vi "HeatFlow Acquire.vi"(0 "HeatFlow HW Tasks in":T4, 1 "HeatFlow HW Cfg":T1, 2 "Runtime":T3, 3 "Last element?":bool) -> (7 "Log Stream":T2, 9 "Display Stream":T2, 10 "error out":errorcluster)   [LabVIEW 2019, in "Acquisition.lvlib"]
doc: "Perform the acquisition. Replace the contents of this diagram with calls to acquisition hardware."
uses:
  Acquisition.lvlib
  HeatFlow HW Tasks.ctl
  Settings/Runtime Conf.ctl
  <extravilib>/ChannelInstances/Stream-var/)Channel.ctl
  HeatFlow HW Cfg.ctl
  HeatFlow Acq Data.ctl
  HeatFlow Acq States.ctl
  <vilib>/DAQmx/read.llb/DAQmx Read (Analog 1D DBL NChan 1Samp).vi
  <vilib>/DAQmx/write.llb/DAQmx Write (Analog 1D DBL NChan 1Samp).vi
  <vilib>/DAQmx/read.llb/DAQmx Read (Analog DBL 1Chan 1Samp).vi
  <extravilib>/ChannelInstances/Stream-var/Write With Abort.vi
  <extravilib>/ChannelInstances/Stream-var/Endpoint.vi
  <vilib>/DAQmx/miscellaneous.llb/DAQmx Fill In Error Info.vi
  <extravilib>/ChannelInstances/Stream-var/)Channel.vi
  <resource>/ChannelSupport/_ChannelSupport/WaitIfNeeded.vi
  <extravilib>/ChannelInstances/Stream-var.lvlib
  Settings/Settings.lvlib
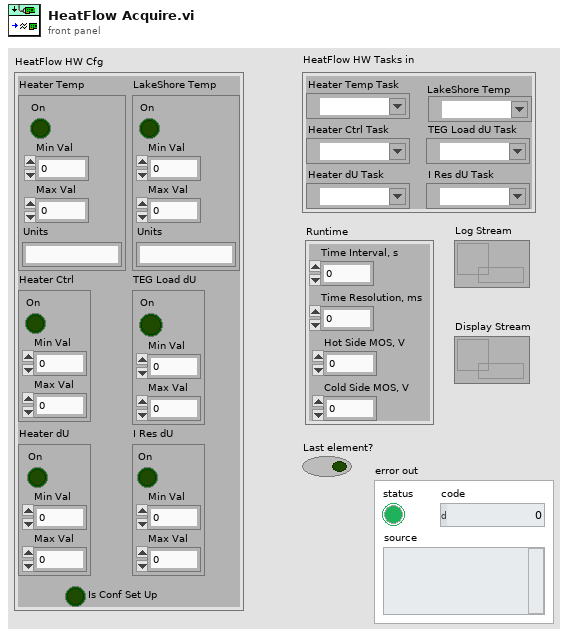
[diagram p1: front panel]
types:
  T1 = typedef "Acquisition.lvlib/HeatFlow HW Cfg.ctl" = cluster{"Heater Temp":cluster{"On":bool, "Min Val":dbl, "Max Val":dbl, "Units":string}, "LakeShore Temp":cluster{"On":bool, "Min Val":dbl, "Max Val":dbl, "Units":string}, "Heater Ctrl":cluster{"On":bool, "Min Val":dbl, "Max Val":dbl}, "TEG Load dU":cluster{"On":bool, "Min Val":dbl, "Max Val":dbl}, "Heater dU":cluster{"On":bool, "Min Val":dbl, "Max Val":dbl}, "I Res dU":cluster{"On":bool, "Min Val":dbl, "Max Val":dbl}, "Is Conf Set Up":bool}
  T2 = typedef "Stream-var.lvlib/)Channel.ctl" = refnum<queue>
  T3 = typedef "Settings.lvlib/Runtime Conf.ctl" = cluster{"Time Interval, s":dbl, "Time Resolution, ms":u32, "Hot Side MOS, V":dbl, "Cold Side MOS, V":dbl}
  T4 = typedef "Acquisition.lvlib/HeatFlow HW Tasks.ctl" = cluster{"Heater Temp Task":refnum<k21>, "Heater Ctrl Task":refnum<k21>, "TEG Load dU Task":refnum<k21>, "Heater dU Task":refnum<k21>, "I Res dU Task":refnum<k21>, "LakeShore Temp":refnum<visa-resource-name>}
  T5 = typedef "Acquisition.lvlib/HeatFlow Acq Data.ctl" = cluster{"Time Stamp":timestamp, "Time Delta":u32, "LakeShore_Temp":cluster{"Tube_T_1":dbl, "Tube_T_2":dbl, "Tube_T_3":dbl, "Tube_T_4":dbl, "Tube_T_5":dbl, "Tube_T_6":dbl, "Tube_T_7":dbl, "Tube_T_8":dbl}, "Heaters":cluster{"I_Res_dU":dbl, "Heater_dU":dbl, "Hot_Side_I":dbl, "Hot_Side_P":dbl, "Cold_Ctrl_U":dbl, "Hot_Ctrl_U":dbl, "Hot_Side_T":dbl, "Cold_Side_T":dbl}, "TEG":cluster{"TEG_Load_dU":dbl, "TEG_Load_R":dbl, "TEG_Load_I":dbl, "TEG_Load_P":dbl, "TEG_eta":dbl, "TEG_dT":dbl, "TEG_U_open":dbl, "TEG_U_Test":dbl, "TEG_R_Test":dbl, "TEG_Rw":dbl}, "LastElement?":bool}
  T6 = typedef "Acquisition.lvlib/HeatFlow Acq States.ctl" = enum16{"Start", "--- Control ---", "HeaterTemp", "DoControl?", "HeaterCtrl", "--- Readings ---", "DoReadings?", "I_Res_dU", "LakeShoreTemp", "Heater_dU", "TEG_Load_dU", "Calculations", "End"}
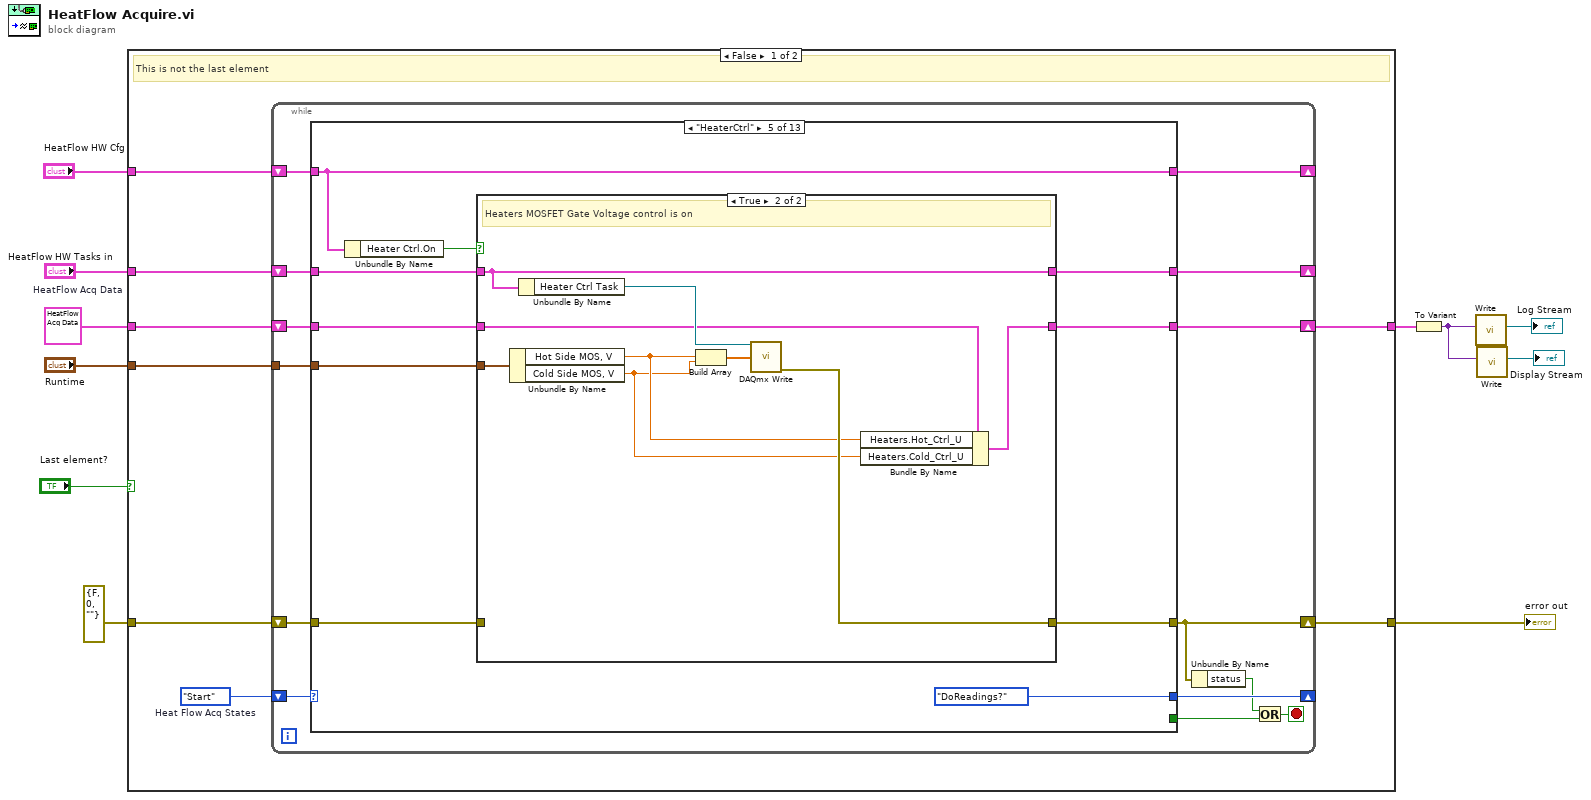
[diagram p0: block diagram]
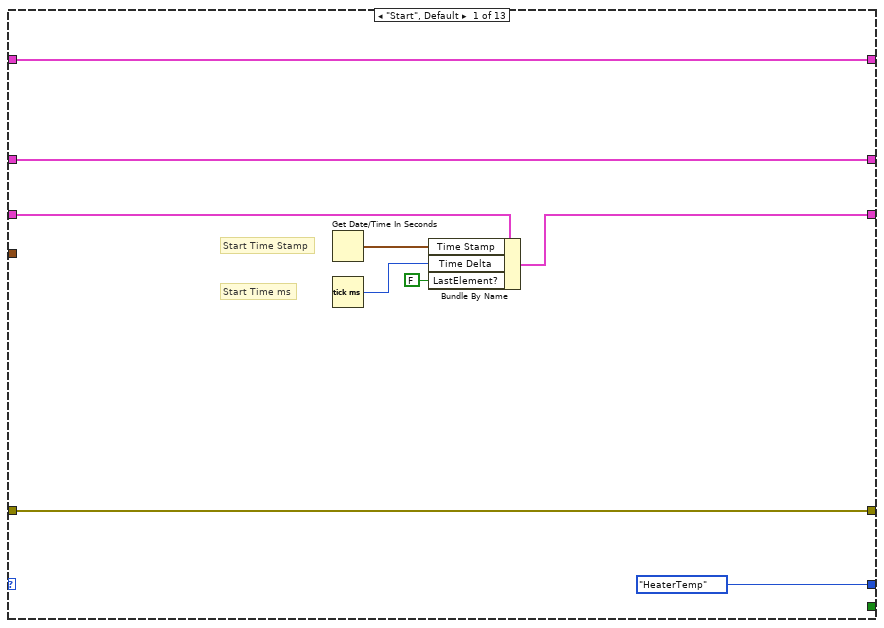
[diagram p2: hidden frame]
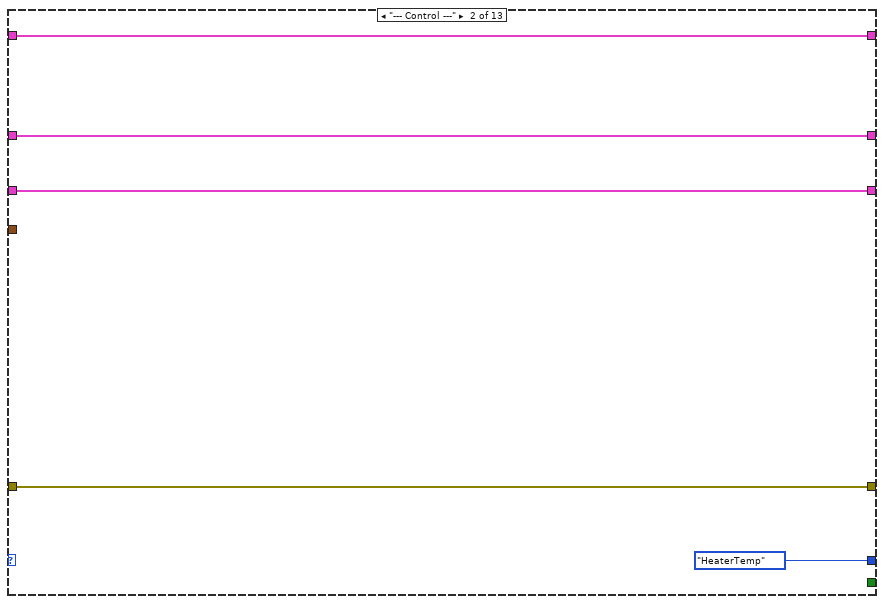
[diagram p3: hidden frame]
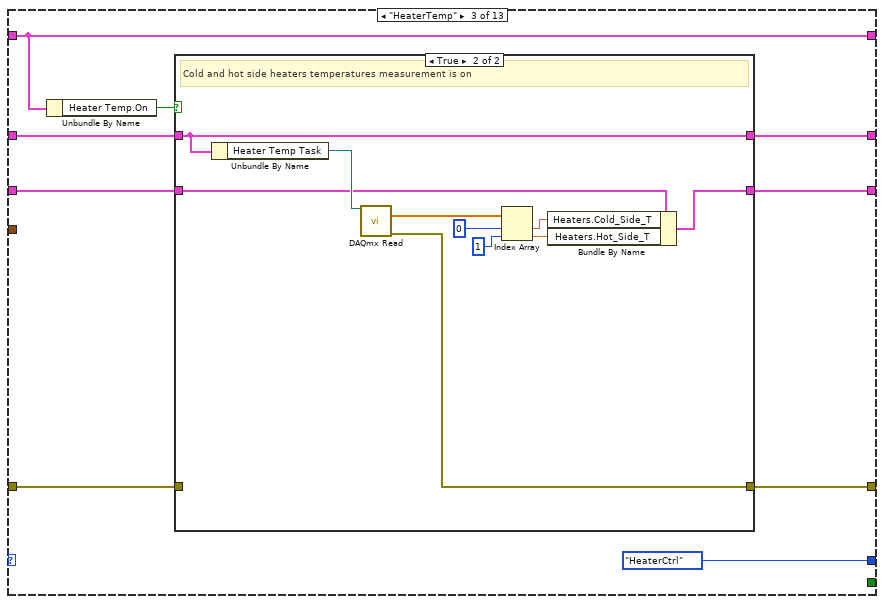
[diagram p4: hidden frame]
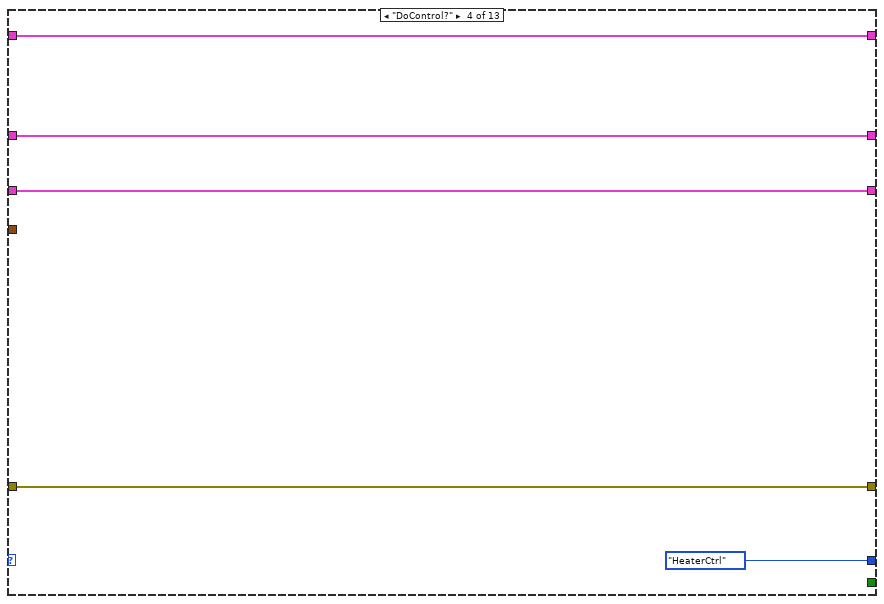
[diagram p6: hidden frame]
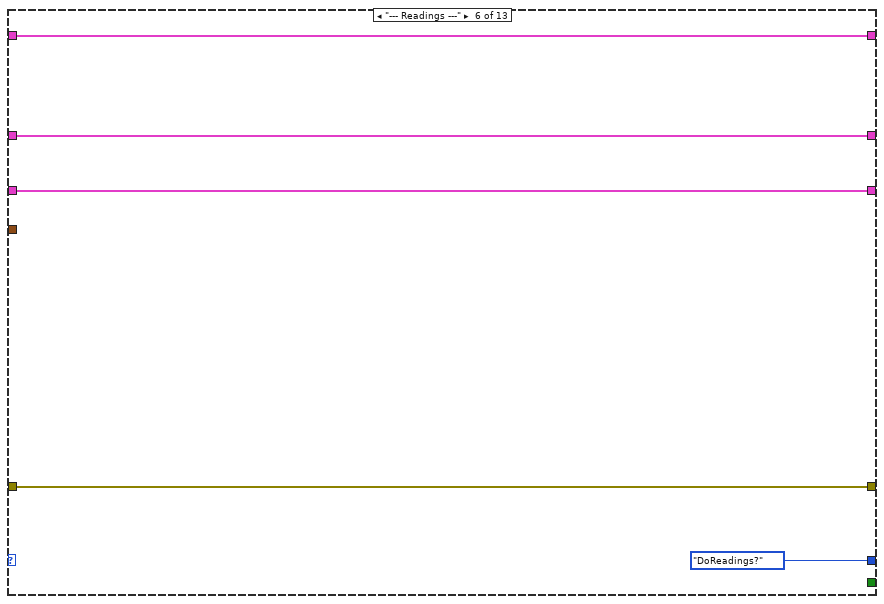
[diagram p8: hidden frame]
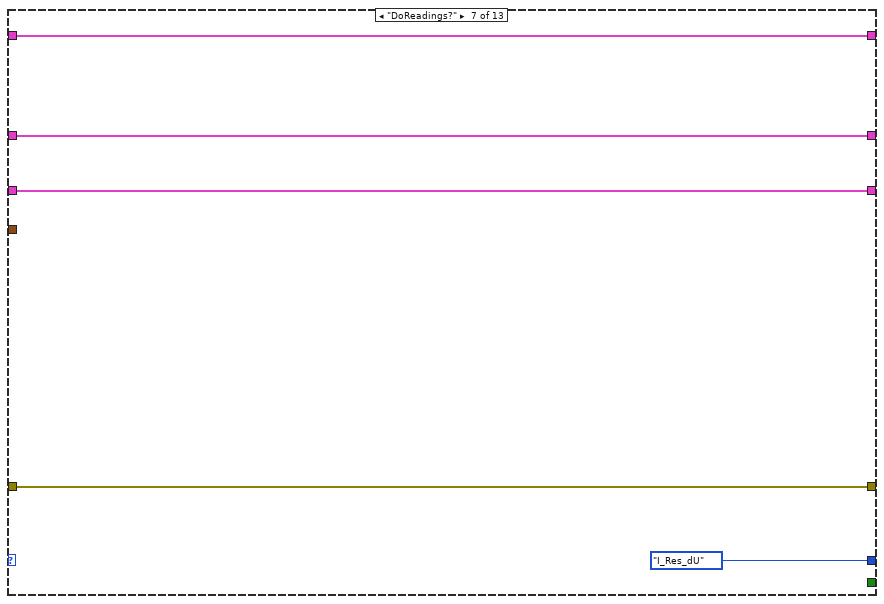
[diagram p9: hidden frame]
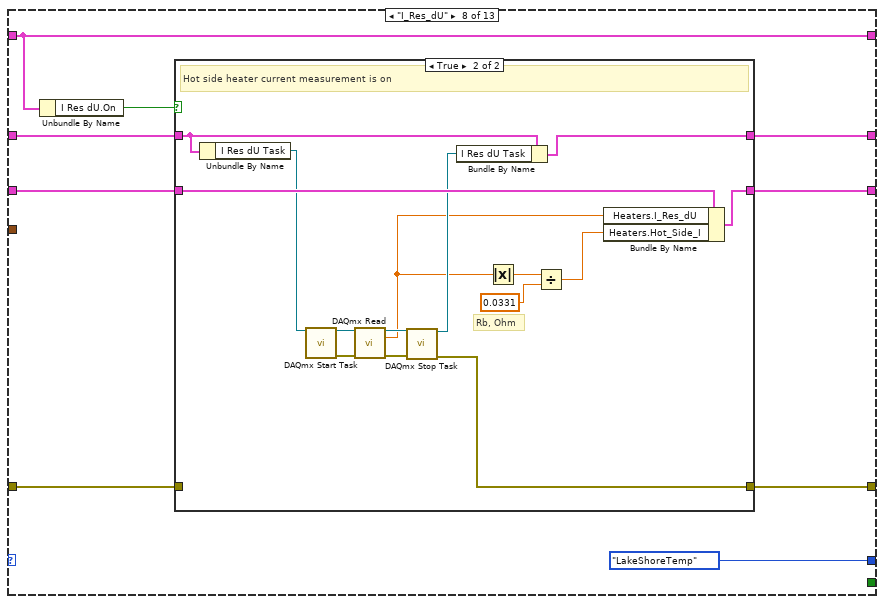
[diagram p10: hidden frame]
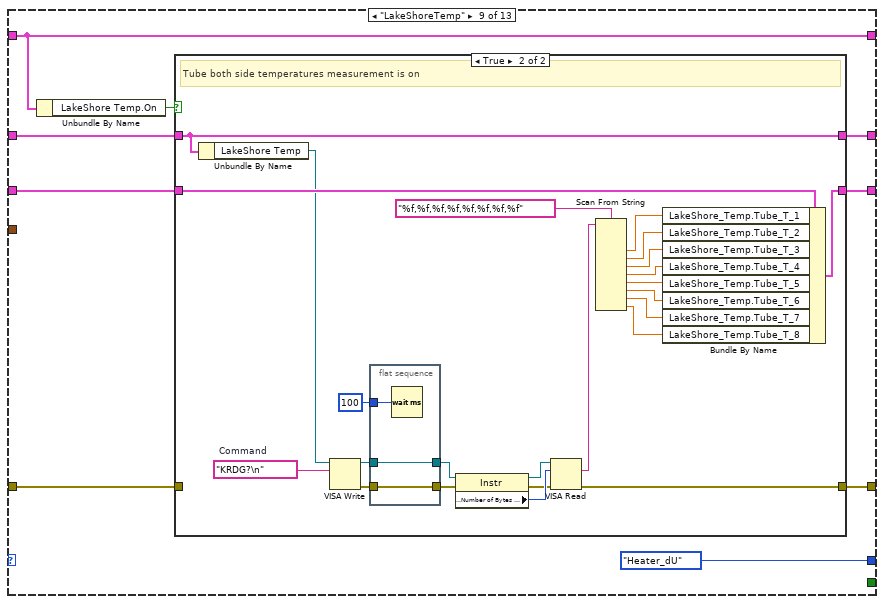
[diagram p12: hidden frame]
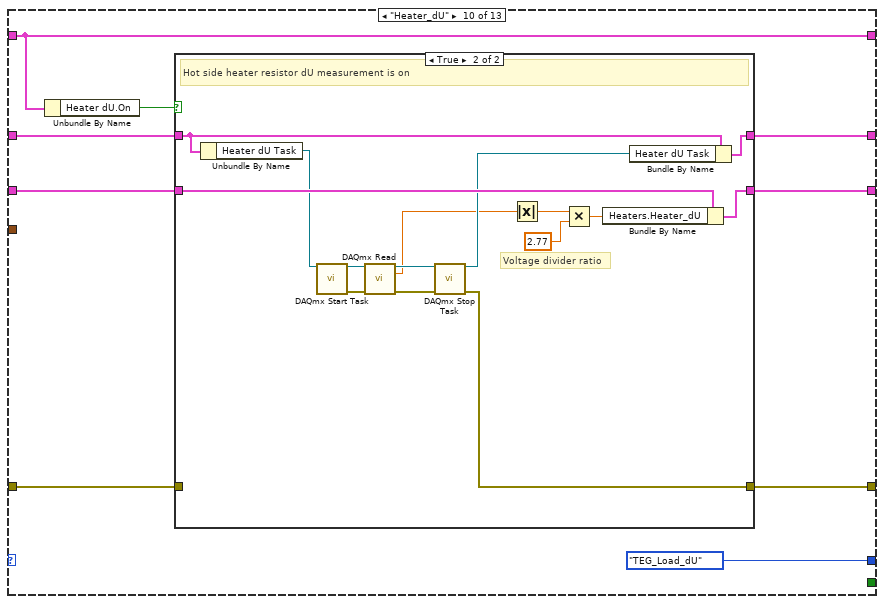
[diagram p14: hidden frame]
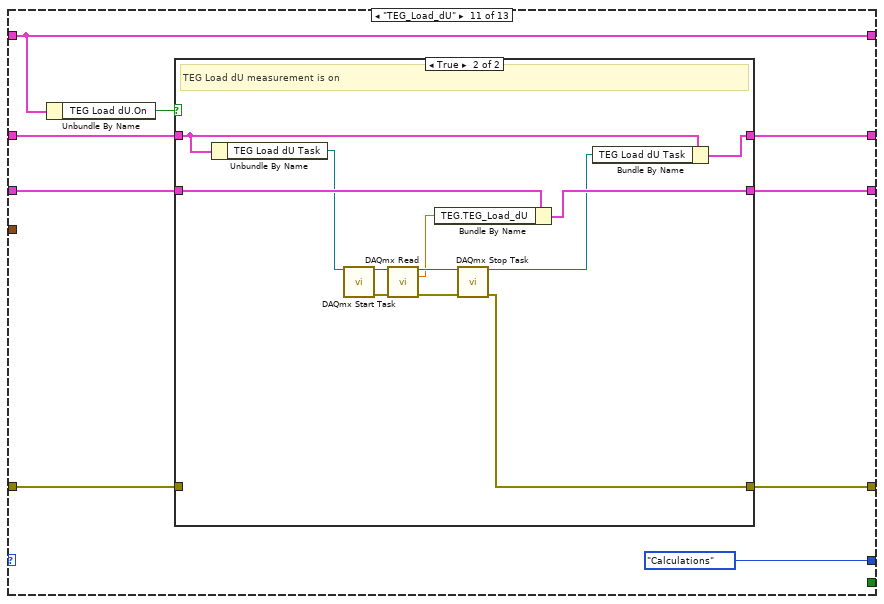
[diagram p16: hidden frame]
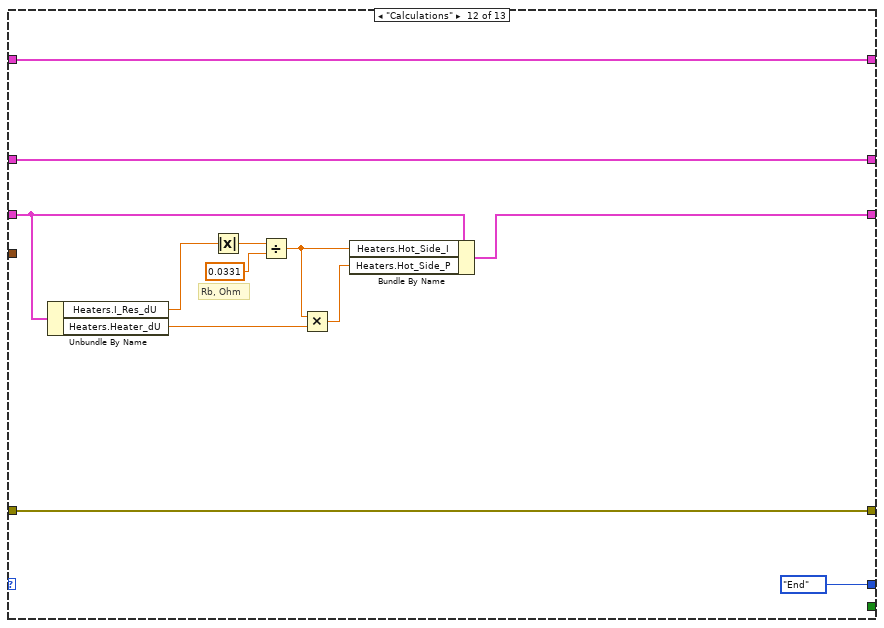
[diagram p18: hidden frame]
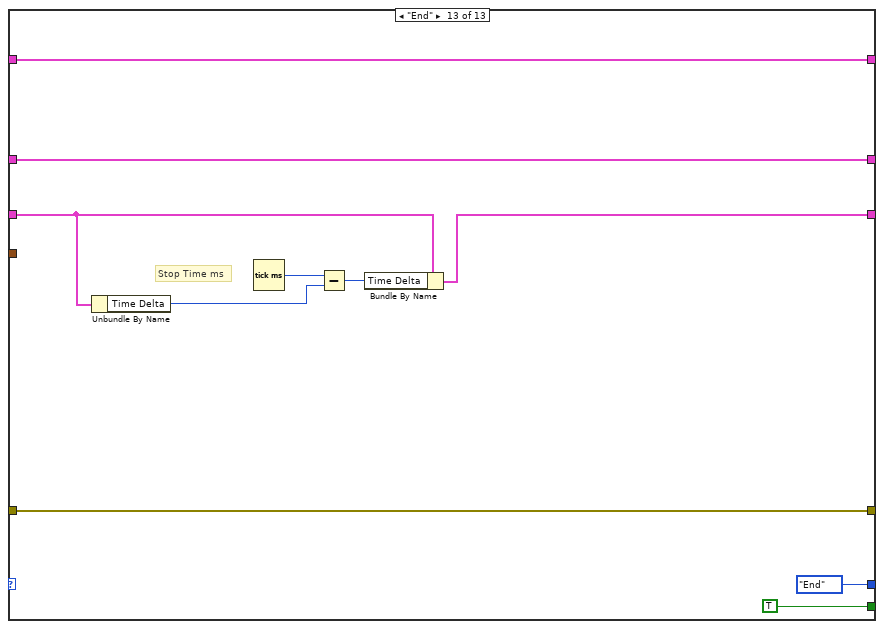
[diagram p19: hidden frame]
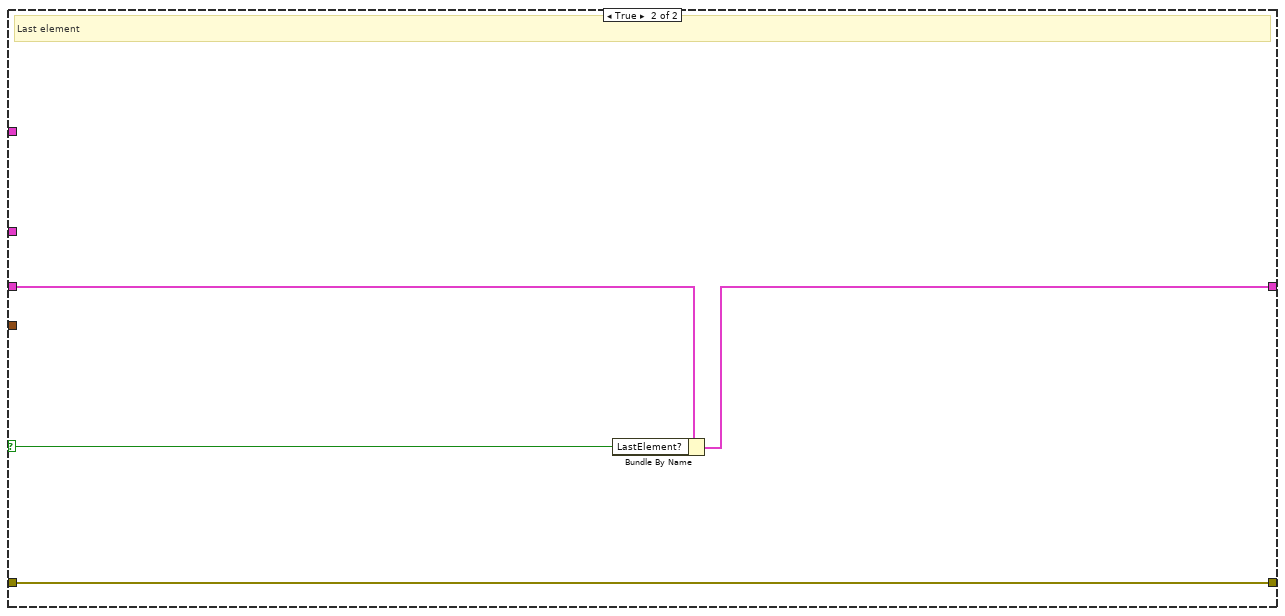
[diagram p20: hidden frame]
diagram:
  w8 = T5 {"Time Stamp"=timestamp(0 s since 1904-01-01), "Time Delta"=0, "LakeShore_Temp"={"Tube_T_1"=0.0, "Tube_T_2"=0.0, "Tube_T_3"=0.0, "Tube_T_4"=0.0, "Tube_T_5"=0.0, "Tube_T_6"=0.0, "Tube_T_7"=0.0, "Tube_T_8"=0.0}, "Heaters"={"I_Res_dU"=0.0, "Heater_dU"=0.0, "Hot_Side_I"=0.0, "Hot_Side_P"=0.0, "Cold_Ctrl_U"=0.0, "Hot_Ctrl_U"=0.0, "Hot_Side_T"=0.0, "Cold_Side_T"=0.0}, "TEG"={"TEG_Load_dU"=0.0, "TEG_Load_R"=0.0, "TEG_Load_I"=0.0, "TEG_Load_P"=0.0, "TEG_eta"=0.0, "TEG_dT"=0.0, "TEG_U_open"=0.0, "TEG_U_Test"=0.0, "TEG_R_Test"=0.0, "TEG_Rw"=0.0}, "LastElement?"=FALSE}  # HeatFlow Acq Data
  n1 = case shown="False" "Last element?" {
    selector: "Last element?" -> [_ w248]
    tunnel: "HeatFlow HW Cfg" -> [w12 _]
    tunnel: "HeatFlow HW Tasks in" -> [w19 _]
    tunnel: errorcluster {"status"=FALSE, "code"=0, "source"=""} ("error out") -> [w18 w246]
    tunnel: [w17 w246] -> w9
    tunnel: w8 -> [w16 w249]
    tunnel: "Runtime" -> [w15 _]
    tunnel: [w14 w247] -> w5
    frame False {
      w13 = HeatFlow_Acq_States."Start"  # Heat Flow Acq States
      # "This is not the last element"
      n2 = while {
        shift-right: [w32] -> _
        shift-left: w13 -> [w33]
        shift-right: [w29] -> _
        shift-left: w19 -> [w31]
        shift-right: [w24] -> w17
        shift-left: w18 -> [w30]
        shift-right: [w27] -> w14
        shift-left: w16 -> [w28]
        tunnel: w15 -> [w22]
        shift-right: [w20] -> _
        shift-left: w12 -> [w21]
        stop <- w25 stop-if-true
        n3 = case shown="\"HeaterCtrl\"" w33 {
          tunnel: [HeatFlow_Acq_States."HeaterTemp" ("Heat Flow States") HeatFlow_Acq_States."HeaterTemp" ("Measurement States") HeatFlow_Acq_States."HeaterCtrl" ("Measurement States") HeatFlow_Acq_States."HeaterCtrl" ("Measurement States") HeatFlow_Acq_States."DoReadings?" ("Measurement States") HeatFlow_Acq_States."DoReadings?" ("Measurement States") HeatFlow_Acq_States."I_Res_dU" ("Measurement States") HeatFlow_Acq_States."LakeShoreTemp" ("Measurement States") HeatFlow_Acq_States."Heater_dU" ("Measurement States") HeatFlow_Acq_States."TEG_Load_dU" ("Measurement States") HeatFlow_Acq_States."Calculations" ("Measurement States") HeatFlow_Acq_States."End" ("Measurement States") HeatFlow_Acq_States."End" ("Measurement States")] -> w32
          tunnel: [_ _ _ _ _ _ _ _ _ _ _ _ TRUE] -> w26
          tunnel: w31 -> [w41 w46 w54 w73 w82 w100 w104 w113 w140 w179 w206 w224 w244]
          tunnel: w30 -> [w36 w44 w53 w71 w81 w98 w102 w112 w139 w178 w205 w227 w241]
          tunnel: [w36 w44 w52 w71 w80 w98 w102 w111 w138 w177 w204 w227 w241] -> w24
          tunnel: [w41 w46 w51 w73 w79 w100 w104 w110 w137 w176 w203 w224 w244] -> w29
          tunnel: w28 -> [w40 w45 w50 w72 w78 w99 w103 w109 w136 w175 w202 w232 w236]
          tunnel: [w37 w45 w49 w72 w77 w99 w103 w108 w135 w174 w201 w228 w243] -> w27
          tunnel: w22 -> [_ _ _ _ w76 _ _ _ _ _ _ _ _]
          tunnel: w21 -> [w35 w47 w48 w74 w75 w101 w105 w107 w134 w173 w200 w225 w237]
          tunnel: [w35 w47 w48 w74 w75 w101 w105 w107 w134 w173 w200 w225 w237] -> w20
          frame "Start", Default {
            # "Start Time ms"
            # "Start Time Stamp"
            n4 = Get Date/Time In Seconds() -> (seconds since 1Jan1904=w39:timestamp)
            n5 = Tick Count (ms)() -> (millisecond timer value=w38:u32)
            n6 = Bundle By Name(cluster=w40, "Time Stamp"=w39, "Time Delta"=w38, "LastElement?"=FALSE) -> (w37:T5)
          }
          frame "--- Control ---" {
          }
          frame "HeaterTemp" {
            n7 = Unbundle By Name(w48) -> ("Heater Temp.On"=w55:bool)
            n8 = case shown="True" w55 {
              tunnel: w54 -> [w59 w68]
              tunnel: w53 -> [w58 _]
              tunnel: [w58 w67] -> w52
              tunnel: [w59 w68] -> w51
              tunnel: w50 -> [w57 w66]
              tunnel: [w57 w65] -> w49
              frame False {
                # "Cold and hot side heaters temperatures measurement is off"
              }
              frame True {
                # "Cold and hot side heaters temperatures measurement is on"
                n9 = Unbundle By Name(w68) -> ("Heater Temp Task"=w69:refnum<k21>)
                n10 = call-poly <vilib>:"DAQmx Read.vi"("task/channels in"=w69) -> ("data"=w64:dbl[], "error out"=w67:errorcluster)  [unwired: 12 in, 1 out]
                n11 = Index Array(array=w64, index #1=0 ("index"), index #2=1 ("index")) -> (element #1=w63:dbl, element #2=w62:dbl)
                n12 = Bundle By Name(cluster=w66, "Heaters.Cold_Side_T"=w63, "Heaters.Hot_Side_T"=w62) -> (w65:T5)
              }
            }
          }
          frame "DoControl?" {
          }
          frame "HeaterCtrl" {
            n13 = Unbundle By Name(w75) -> ("Heater Ctrl.On"=w83:bool)
            n14 = case shown="True" w83 {
              tunnel: w82 -> [w87 w95]
              tunnel: w81 -> [w86 _]
              tunnel: [w86 w94] -> w80
              tunnel: [w87 w95] -> w79
              tunnel: w78 -> [w85 w93]
              tunnel: [w85 w91] -> w77
              tunnel: w76 -> [_ w90]
              frame False {
                # "Heaters MOSFET Gate Voltage control is off"
              }
              frame True {
                # "Heaters MOSFET Gate Voltage control is on"
                n15 = Unbundle By Name(w90) -> ("Hot Side MOS, V"=w89:dbl, "Cold Side MOS, V"=w88:dbl)
                n16 = Unbundle By Name(w95) -> ("Heater Ctrl Task"=w96:refnum<k21>)
                n17 = Build Array(w89, w88) -> (w92:dbl[])
                n18 = call-poly <vilib>:"DAQmx Write.vi"("task/channels in"=w96, "data"=w92) -> ("error out"=w94:errorcluster)  [unwired: 11 in, 2 out]
                n19 = Bundle By Name(cluster=w93, "Heaters.Hot_Ctrl_U"=w89, "Heaters.Cold_Ctrl_U"=w88) -> (w91:T5)
              }
            }
          }
          frame "--- Readings ---" {
          }
          frame "DoReadings?" {
          }
          frame "I_Res_dU" {
            n20 = Unbundle By Name(w107) -> ("I Res dU.On"=w114:bool)
            n21 = case shown="True" w114 {
              tunnel: w113 -> [w118 w125]
              tunnel: w112 -> [w117 _]
              tunnel: [w117 w127] -> w111
              tunnel: [w118 w123] -> w110
              tunnel: w109 -> [w116 w133]
              tunnel: [w116 w132] -> w108
              frame False {
                # "Hot side heater current measurement is off"
              }
              frame True {
                # "Rb, Ohm"
                # "Hot side heater current measurement is on"
                n22 = Unbundle By Name(w125) -> ("I Res dU Task"=w130:refnum<k21>)
                n23 = call <vilib>:"DAQmx Start Task.vi"("task/channels in"=w130) -> ("task out"=w129:refnum<k21>, "error out"=w131:errorcluster)  [unwired: 13 in]
                n24 = call-poly <vilib>:"DAQmx Read.vi"("task/channels in"=w129, "error in"=w131) -> ("task out"=w126:refnum<k21>, "data"=w119:dbl, "error out"=w128:errorcluster)  [unwired: 11 in]
                n25 = call <vilib>:"DAQmx Stop Task.vi"("task/channels in"=w126, "error in"=w128) -> ("task out"=w124:refnum<k21>, "error out"=w127:errorcluster)  [unwired: 12 in]
                n26 = Bundle By Name(cluster=w125, "I Res dU Task"=w124) -> (w123:T4)
                n27 = Absolute Value(x=w119) -> (abs(x)=w122:dbl)
                n28 = Divide(x=w122, y=0.0331) -> (x/y=w120:dbl)
                n29 = Bundle By Name(cluster=w133, "Heaters.I_Res_dU"=w119, "Heaters.Hot_Side_I"=w120) -> (w132:T5)
              }
            }
          }
          frame "LakeShoreTemp" {
            n30 = Unbundle By Name(w134) -> ("LakeShore Temp.On"=w141:bool)
            n31 = case shown="True" w141 {
              tunnel: w140 -> [w145 w169]
              tunnel: w139 -> [w144 _]
              tunnel: [w144 w146] -> w138
              tunnel: [w145 w169] -> w137
              tunnel: w136 -> [w143 w168]
              tunnel: [w143 w167] -> w135
              frame False {
                # "Tube both side temperatures measurement is off"
              }
              frame True {
                w163 = "KRDG?\n"  # Command
                # "Tube both side temperatures measurement is on"
                n32 = Unbundle By Name(w169) -> ("LakeShore Temp"=w147:refnum<visa-resource-name>)
                n33 = VISA Write(VISA resource name=w147, write buffer=w163) -> (VISA resource name out=w160:refnum<visa-resource-name>, error out=w158:errorcluster)  [unwired: 1 in, 1 out]
                n34 = flat-sequence {
                  tunnel: w158 -> [w171]
                  tunnel: [w171] -> w159
                  tunnel: w160 -> [w170]
                  tunnel: [w170] -> w161
                  tunnel: u32 100 ("delay before read (ms)") -> [w172]
                  frame #0 {
                    n35 = Wait (ms)(milliseconds to wait=w172) -> ()  [unwired: 1 out]
                  }
                }
                n36 = property class="Instr"(reference=w161, error in=w159) -> (reference out=w164:refnum<visa-resource-name>, error out=w165:errorcluster, "Serial Settings:Number of Bytes at Serial Port"=w166:u32)
                n37 = VISA Read(VISA resource name=w164, byte count=w166, error in (no error)=w165) -> (read buffer=w156:string, error out=w146:errorcluster)  [unwired: 2 out]
                n38 = Scan From String(format string="%f,%f,%f,%f,%f,%f,%f,%f", input string=w156) -> (output 1=w148:dbl, output 2=w149:dbl, output 3=w150:dbl, output 4=w152:dbl, output 5=w153:dbl, output 6=w154:dbl, output 7=w151:dbl, output 8=w155:dbl)  [unwired: 10 in, 3 out]
                n39 = Bundle By Name(cluster=w168, "LakeShore_Temp.Tube_T_1"=w148, "LakeShore_Temp.Tube_T_2"=w149, "LakeShore_Temp.Tube_T_3"=w150, "LakeShore_Temp.Tube_T_4"=w152, "LakeShore_Temp.Tube_T_5"=w153, "LakeShore_Temp.Tube_T_6"=w154, "LakeShore_Temp.Tube_T_7"=w151, "LakeShore_Temp.Tube_T_8"=w155) -> (w167:T5)
              }
            }
          }
          frame "Heater_dU" {
            n40 = Unbundle By Name(w173) -> ("Heater dU.On"=w180:bool)
            n41 = case shown="True" w180 {
              tunnel: w179 -> [w184 w192]
              tunnel: w178 -> [w183 _]
              tunnel: [w183 w189] -> w177
              tunnel: [w184 w190] -> w176
              tunnel: w175 -> [w182 w199]
              tunnel: [w182 w198] -> w174
              frame False {
                # "Hot side heater resistor dU measurement is off"
              }
              frame True {
                # "Voltage divider ratio"
                # "Hot side heater resistor dU measurement is on"
                n42 = Unbundle By Name(w192) -> ("Heater dU Task"=w193:refnum<k21>)
                n43 = call <vilib>:"DAQmx Start Task.vi"("task/channels in"=w193) -> ("task out"=w197:refnum<k21>, "error out"=w196:errorcluster)  [unwired: 13 in]
                n44 = call-poly <vilib>:"DAQmx Read.vi"("task/channels in"=w197, "error in"=w196) -> ("task out"=w195:refnum<k21>, "data"=w185:dbl, "error out"=w194:errorcluster)  [unwired: 11 in]
                n45 = call <vilib>:"DAQmx Stop Task.vi"("task/channels in"=w195, "error in"=w194) -> ("task out"=w191:refnum<k21>, "error out"=w189:errorcluster)  [unwired: 12 in]
                n46 = Absolute Value(x=w185) -> (abs(x)=w187:dbl)
                n47 = Multiply(x=w187, y=2.77) -> (x*y=w186:dbl)
                n48 = Bundle By Name(cluster=w199, "Heaters.Heater_dU"=w186) -> (w198:T5)
                n49 = Bundle By Name(cluster=w192, "Heater dU Task"=w191) -> (w190:T4)
              }
            }
          }
          frame "TEG_Load_dU" {
            n50 = Unbundle By Name(w200) -> ("TEG Load dU.On"=w207:bool)
            n51 = case shown="True" w207 {
              tunnel: w206 -> [w211 w217]
              tunnel: w205 -> [w210 _]
              tunnel: [w210 w213] -> w204
              tunnel: [w211 w216] -> w203
              tunnel: w202 -> [w209 w223]
              tunnel: [w209 w222] -> w201
              frame False {
                # "TEG Load dU measurement is off"
              }
              frame True {
                # "TEG Load dU measurement is on"
                n52 = Unbundle By Name(w217) -> ("TEG Load dU Task"=w212:refnum<k21>)
                n53 = call <vilib>:"DAQmx Start Task.vi"("task/channels in"=w212) -> ("task out"=w221:refnum<k21>, "error out"=w220:errorcluster)  [unwired: 13 in]
                n54 = call-poly <vilib>:"DAQmx Read.vi"("task/channels in"=w221, "error in"=w220) -> ("task out"=w219:refnum<k21>, "data"=w215:dbl, "error out"=w218:errorcluster)  [unwired: 11 in]
                n55 = Bundle By Name(cluster=w223, "TEG.TEG_Load_dU"=w215) -> (w222:T5)
                n56 = call <vilib>:"DAQmx Stop Task.vi"("task/channels in"=w219, "error in"=w218) -> ("task out"=w214:refnum<k21>, "error out"=w213:errorcluster)  [unwired: 12 in]
                n57 = Bundle By Name(cluster=w217, "TEG Load dU Task"=w214) -> (w216:T4)
              }
            }
          }
          frame "Calculations" {
            # "Rb, Ohm"
            n58 = Unbundle By Name(w232) -> ("Heaters.I_Res_dU"=w233:dbl, "Heaters.Heater_dU"=w231:dbl)
            n59 = Absolute Value(x=w233) -> (abs(x)=w235:dbl)
            n60 = Divide(x=w235, y=0.0331) -> (x/y=w229:dbl)
            n61 = Multiply(x=w229, y=w231) -> (x*y=w230:dbl)
            n62 = Bundle By Name(cluster=w232, "Heaters.Hot_Side_I"=w229, "Heaters.Hot_Side_P"=w230) -> (w228:T5)
          }
          frame "End" {
            # "Stop Time ms"
            n63 = Unbundle By Name(w236) -> ("Time Delta"=w239:u32)
            n64 = Tick Count (ms)() -> (millisecond timer value=w240:u32)
            n65 = Subtract(x=w240, y=w239) -> (x-y=w238:u32)
            n66 = Bundle By Name(cluster=w236, "Time Delta"=w238) -> (w243:T5)
          }
        }
        n67 = Unbundle By Name(w24) -> ("status"=w23:bool)
        n68 = Or(x=w23, y=w26) -> (x .or. y?=w25:bool)
      }
    }
    frame True {
      # "Last element"
      n69 = Bundle By Name(cluster=w249, "LastElement?"=w248) -> (w247:T5)
    }
  }
  "error out" <- w9
  n70 = To Variant(anything=w5) -> (Variant=w4:variant)
  n71 = call <extravilib>:"Write.vi"("element"=w4) -> ("channel"=→"Log Stream":T2)  [unwired: 8 in, 2 out]
  n72 = call <extravilib>:"Write.vi"("element"=w4) -> ("channel"=→"Display Stream":T2)  [unwired: 8 in, 2 out]
